vi "Main.vi"() -> ()   [LabVIEW 2017]
panel:
  in  "Sensors Mode":bool
  out "T5":dbl(slide) scale=0.0..150.0
  out "T7":dbl(slide) scale=0.0..150.0
  out "T3":dbl(slide) scale=0.0..150.0
  out "T8":dbl(slide) scale=0.0..150.0
  out "T1":dbl(slide) scale=0.0..150.0
  out "T9":dbl(slide) scale=0.0..150.0
  out "T2":dbl(slide) scale=0.0..150.0
  out "T4":dbl(slide) scale=0.0..150.0
  out "T6":dbl(slide) scale=0.0..150.0
  out "Heater Power":dbl caption="Heater Power P [W]" format="%#.2f"
  out "Heater Temperature":dbl(slide) scale=0.0..250.0
  out "NI2":tag
  out "NI1":tag
  out "Tab Control":enum32{"Page 1", "Page 2"}(tab)
  in  "reset":bool
  in  "Play Button":bool
  out "sec":i16
  out "min":i16
  out "hr":i16
  out "Ky [W/m.K]":dbl
  out "Ks [W/m.K]":dbl
  out "K7-8 [W/m.K]":dbl
  out "K6-7 [W/m.K]":dbl
  out "K5-6 [W/m.K]":dbl
  out "K4-5 [W/m.K]":dbl
  out "K3-4 [W/m.K]":dbl
  out "K2-3 [W/m.K]":dbl
  in  "Exit":bool
  out "X 7 mm":dbl
  out "X 8 mm":dbl
  out "X 9 mm":dbl
  out "X 6 mm":dbl
  out "X 5 mm":dbl
  out "X 4 mm":dbl
  out "X 3 mm":dbl
  out "X 2 mm":dbl
  out "X 1 mm":dbl
  out "K1-2 [W/m.K]":dbl
  out "Heater Temperature T0 [C]":dbl(slide) scale=0.0..250.0
  out "T5 C":dbl(slide) scale=0.0..150.0
  out "T6 C":dbl(slide) scale=0.0..150.0
  out "T4 C":dbl(slide) scale=0.0..150.0
  out "T9 C":dbl(slide) scale=0.0..150.0
  out "T8 C":dbl(slide) scale=0.0..150.0
  out "T7 C":dbl(slide) scale=0.0..150.0
  out "T3 C":dbl(slide) scale=0.0..150.0
  out "T2 C":dbl(slide) scale=0.0..150.0
  out "T1 C":dbl(slide) scale=0.0..150.0
  out "Heater Power linear":dbl caption="Heater Power P [W]" format="%#.2f"
  out "Diameter d [mm]":dbl
  in  "Material Select":string(combo)
  out "Linear Temperature Profile":cluster{"Ramp Pattern":dbl[], dbl[]}[](graph)
  in  "Start Linear":bool
  in  "To Radial":bool
  in  "Save Linear Curve":bool
  in  "Clear Linear Graph":bool
  in  "reset 2":bool
  out "hr 2":i16
  out "min 2":i16
  out "sec 2":i16
  in  "Play Button 2":bool
  out "T45":dbl caption="T45 C" format="%#_5g"
  out "T34":dbl caption="T34 C" format="%#_5g"
  out "T23":dbl caption="T23 C" format="%#_5g"
  out "T12":dbl caption="T12 C" format="%#_5g"
  in  "Exit 2":bool
  out "Thermal Conductivity K [W/m.K]":dbl
  out "T6r":dbl caption="T9 C" format="%#_5g"
  out "T5r":dbl caption="T8 C" format="%#_5g"
  out "T4r":dbl caption="T7 C" format="%#_5g"
  out "T3r":dbl caption="T3 C" format="%#_5g"
  out "T2r":dbl caption="T2 C" format="%#_5g"
  out "T1r":dbl caption="T1 C" format="%#_5g"
  out "Heater Temperature [C]":dbl format="%#_5g"
  out "r1":dbl caption="r1 mm" format="%#_5g"
  out "r2":dbl caption="r2 mm" format="%#_5g"
  out "r3":dbl caption="r3 mm" format="%#_5g"
  out "r4":dbl caption="r4 mm" format="%#_5g"
  out "r5":dbl caption="r5 mm" format="%#_5g"
  out "r6":dbl caption="r6 mm" format="%#_5g"
  out "Radial Temperature Profile":cluster{"Ramp Pattern":dbl[], dbl[]}[](graph)
  in  "To Linear":bool
  in  "Clear Radial Graph":bool
  in  "Save Radial Curve":bool
  out "ri [mm]":dbl caption="Inner Radius ri [mm]"
  out "ro [mm]":dbl caption="Outer Radius ro [mm]"
  out "Disk Thickness [mm]":dbl caption="Disk thinkness t [mm]"
  out "Heater Power rad":dbl caption="Heater Power P [W]"
  in  "Start radial":bool
  # "9"
  # "6"
  # ":"
  # ":"
  # "Linear Experment"
  # "Cooler or heat sink"
  # "Radial Experment"
  # ":"
  # ":"
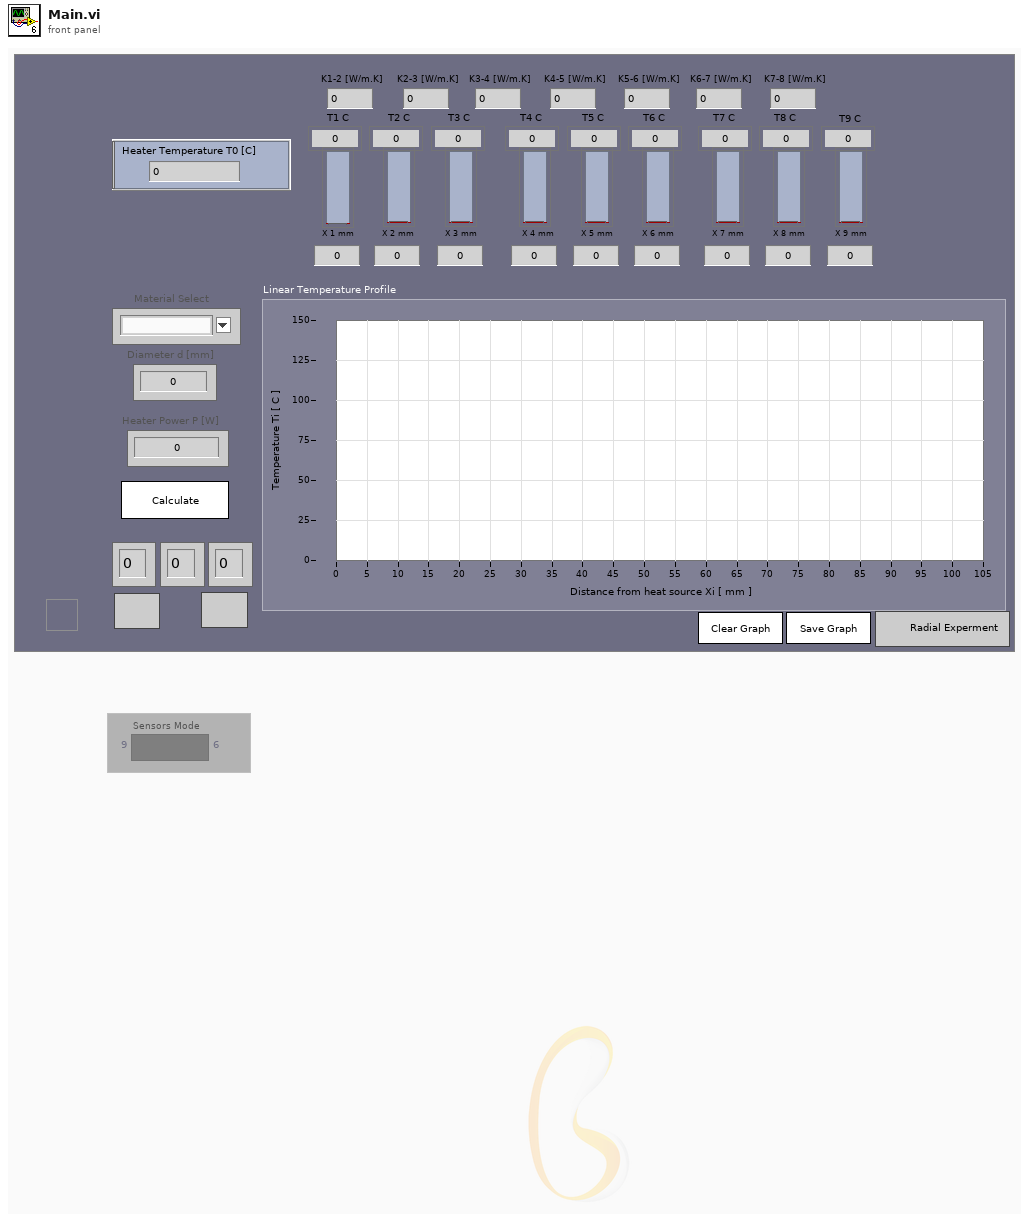
[diagram p1: front panel]
types:
  T1 = enum8{"Enabled", "Disabled", "Disabled and Grayed Out"}
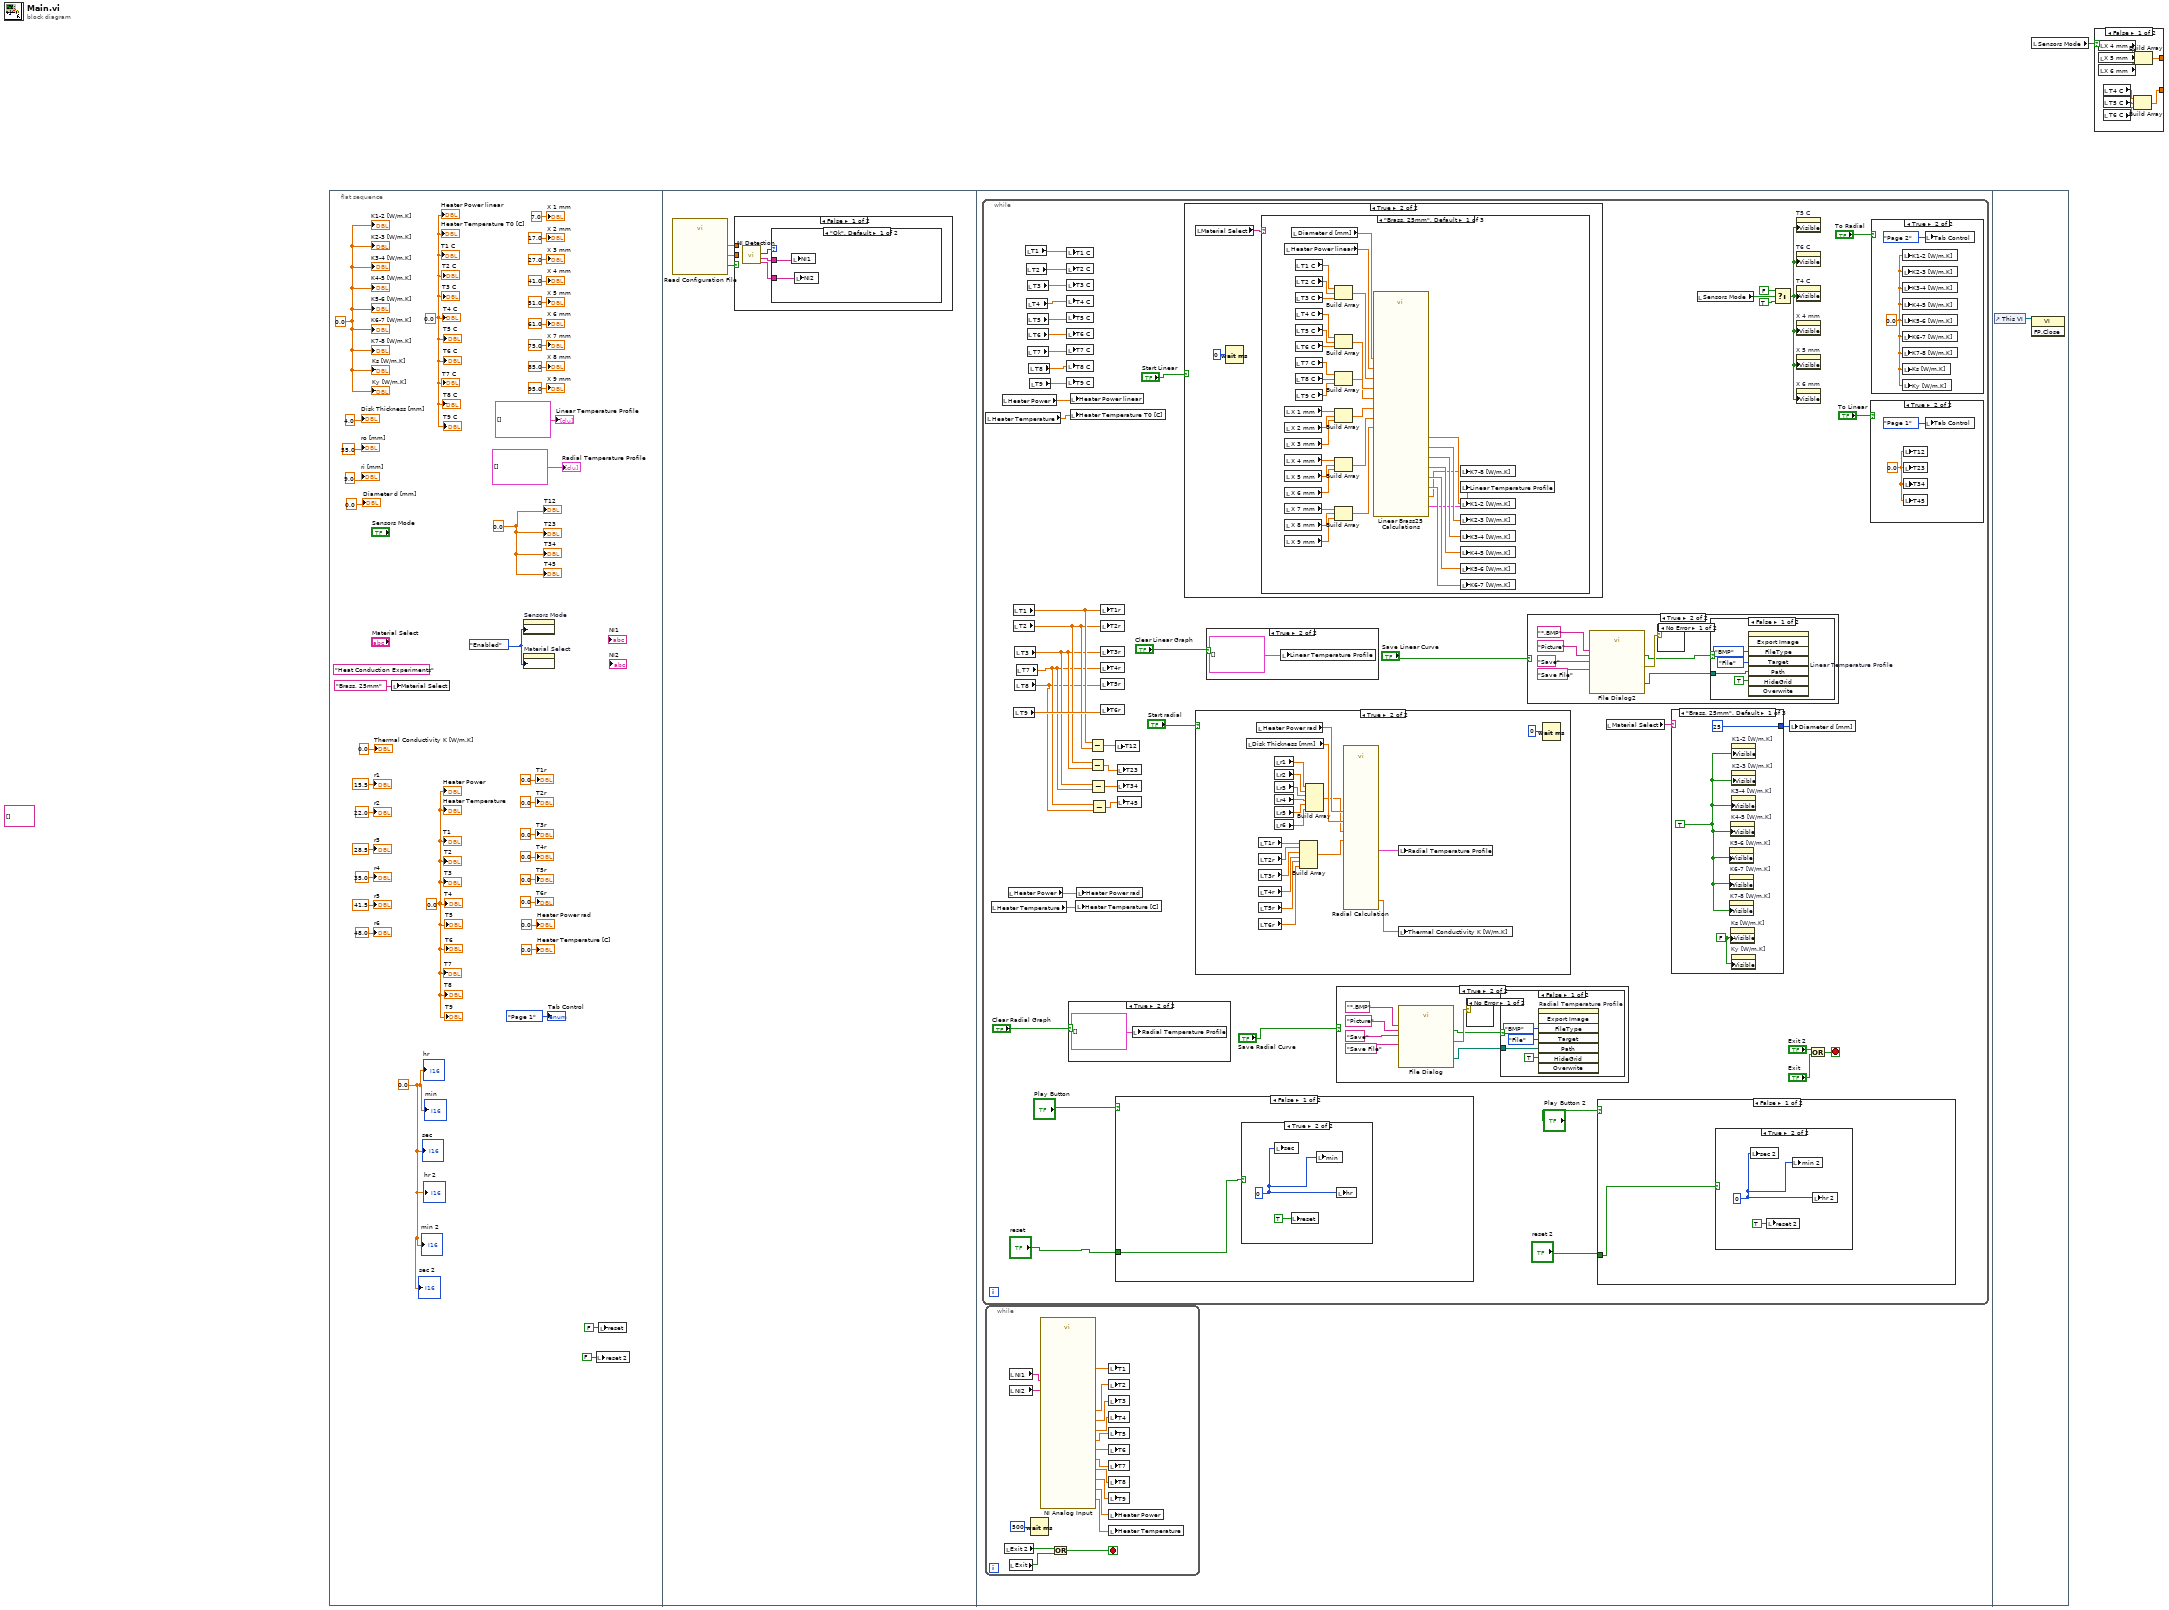
[diagram p0: block diagram]
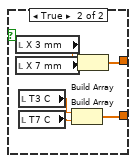
[diagram p2: hidden frame]
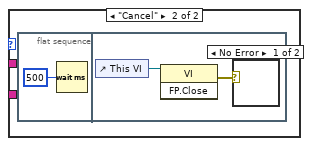
[diagram p3: hidden frame]
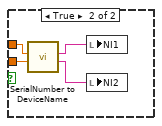
[diagram p5: hidden frame]
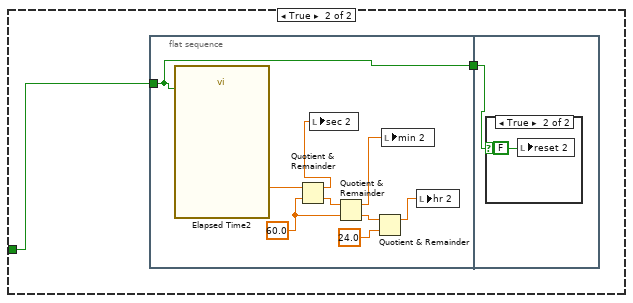
[diagram p7: hidden frame]
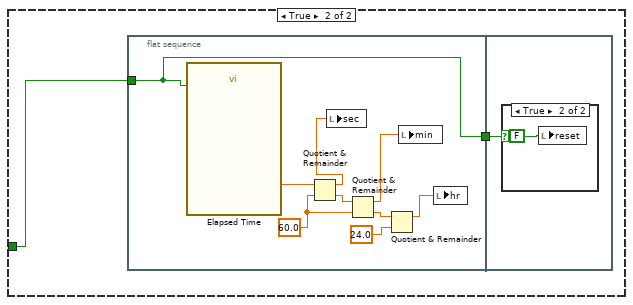
[diagram p10: hidden frame]
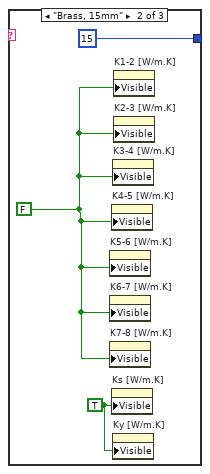
[diagram p14: hidden frame]
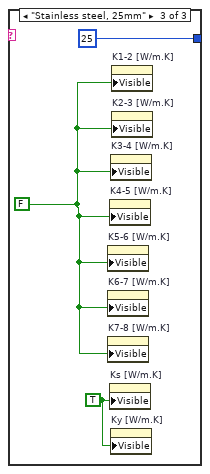
[diagram p15: hidden frame]
diagram:
  (unwired) string[][] [] ("Temperature Table 2")
  n1 = flat-sequence {
    frame #0 {
      w4 = 0.0 ("K")
      w6 = 0.0 ("K1-2 [W/m.K]")
      w5 = 0.0 ("k1- 2")
      w7 = 0.0 ("X1")
      w12 = 0.0 ("X1")
      w36 = T1."Enabled" ("Disabled")
      (unwired) "Heat Conduction Experiments" ("String")
      n2 = local write "Material Select"("Brass, 25mm" ("Material Select")) -> ()
      n3 = property on="Sensors Mode" class="Bool (strict)"("DisabledEnum"=w36) -> ()  [unwired: 2 in, 2 out]
      n4 = property on="Material Select" class="CmbBox"("DisabledEnum"=w36) -> ()  [unwired: 2 in, 2 out]
      n5 = local write "reset 2"(FALSE ("reset 2")) -> ()
      n6 = local write "reset"(FALSE ("reset")) -> ()
      "r3" <- 28.5 ("r3")
      "r2" <- 22.0 ("r2")
      "r1" <- 15.5 ("r1")
      "r4" <- 35.0 ("r4")
      "r5" <- 41.5 ("r5")
      "r6" <- 48.0 ("r6")
      "Heater Power rad" <- 0.0 ("Heater Power rad")
      "Heater Temperature [C]" <- 0.0 ("Heater Temperature")
      "Diameter d [mm]" <- 0.0 ("Diameter d [mm]")
      "ro [mm]" <- 55.0 ("Diameter [mm] radial")
      "Disk Thickness [mm]" <- 4.0 ("Distance [mm] radial")
      "ri [mm]" <- 9.0 ("ri [mm]")
      "X 1 mm" <- 7.0 ("X 1")
      "X 2 mm" <- 17.0 ("X 2")
      "X 3 mm" <- 27.0 ("X 3")
      "X 4 mm" <- 41.0 ("X 4")
      "X 5 mm" <- 51.0 ("X 5")
      "X 6 mm" <- 61.0 ("X 6")
      "X 7 mm" <- 75.0 ("X 7")
      "X 8 mm" <- 85.0 ("X 8")
      "X 9 mm" <- 95.0 ("X 9")
      "Radial Temperature Profile" <- cluster{"Ramp Pattern":dbl[], dbl[]}[] [] ("Temperature Graph radial")
      "Linear Temperature Profile" <- cluster{"Ramp Pattern":dbl[], dbl[]}[] [] ("Linear Temperature Profile")
      "T1r" <- 0.0 ("T1")
      "T2r" <- 0.0 ("T2")
      "T3r" <- 0.0 ("T3")
      "T4r" <- 0.0 ("T4")
      "T5r" <- 0.0 ("T5")
      "T6r" <- 0.0 ("T6")
      "T5 C" <- w12
      "T7 C" <- w12
      "T3 C" <- w12
      "T8 C" <- w12
      "T1 C" <- w12
      "T9 C" <- w12
      "T2 C" <- w12
      "T4 C" <- w12
      "T6 C" <- w12
      "Heater Power linear" <- w12
      "Heater Temperature T0 [C]" <- w12
      "Thermal Conductivity K [W/m.K]" <- 0.0 ("Thermal Conductivity K [W/m.K]")
      "Tab Control" <- enum32{"Page 1", "Page 2"}."Page 1" ("Tab Control")
      "T5" <- w7
      "T7" <- w7
      "T3" <- w7
      "T8" <- w7
      "T1" <- w7
      "T9" <- w7
      "T2" <- w7
      "T4" <- w7
      "T6" <- w7
      "Heater Power" <- w7
      "Heater Temperature" <- w7
      "K2-3 [W/m.K]" <- w6
      "K3-4 [W/m.K]" <- w6
      "K4-5 [W/m.K]" <- w6
      "K5-6 [W/m.K]" <- w6
      "K6-7 [W/m.K]" <- w6
      "K7-8 [W/m.K]" <- w6
      "Ks [W/m.K]" <- w6
      "Ky [W/m.K]" <- w6
      "K1-2 [W/m.K]" <- w6
      "T12" <- w5
      "T23" <- w5
      "T34" <- w5
      "T45" <- w5
      "sec" <- w4
      "min" <- w4
      "hr" <- w4
      "hr 2" <- w4
      "min 2" <- w4
      "sec 2" <- w4
    }
    frame #1 {
      n7 = call "Read Configuration File.vi"() -> ("Serial Numbers Found"=w42:bool, "NI1"=w44:dbl, "NI2"=w43:dbl)  [unwired: 13 in]
      n8 = case shown="False" w42 {
        tunnel: w43 -> [_ w56]
        tunnel: w44 -> [_ w55]
        frame False {
          n9 = call "NI Detection.vi"() -> ("NI 2"=w45:tag, "NI 1"=w46:tag, "Ok/Cancel"=w47:enum16{"Ok", "Cancel"})  [unwired: 8 in]
          n10 = case shown="\"Ok\", Default" w47 {
            tunnel: w46 -> [w49 _]
            tunnel: w45 -> [w48 _]
            frame "Ok", Default {
              n11 = local write "NI1"(w49) -> ()
              n12 = local write "NI2"(w48) -> ()
            }
            frame "Cancel" {
              n13 = flat-sequence {
                frame #0 {
                  n14 = Wait (ms)(milliseconds to wait=u32 500) -> ()  [unwired: 1 out]
                }
                frame #1 {
                  n15 = control-ref of="This VI"() -> (w52:refnum<vi>)
                  n16 = invoke class="VI" method="FP.Close"(reference=w52) -> (error out=w51:errorcluster)  [unwired: 2 in, 2 out]
                  n17 = case shown="No Error" w51 {
                    frame No Error {
                    }
                    frame Error {
                    }
                  }
                }
              }
            }
          }
        }
        frame True {
          n18 = call "SerialNumber to DeviceName.vi"("NI2 Serial Number"=w56, "NI1 Serial Number"=w55) -> ("NI2 Device Name"=w53:tag, "NI1 Device Name"=w54:tag)  [unwired: 8 in]
          n19 = local write "NI1"(w54) -> ()
          n20 = local write "NI2"(w53) -> ()
        }
      }
    }
    frame #2 {
      n21 = while {
        stop <- w103 stop-if-true
        n22 = local read "Heater Temperature"() -> (w102:dbl)
        n23 = local read "Heater Temperature"() -> (w89:dbl)
        n24 = local read "Heater Power"() -> (w101:dbl)
        n25 = local read "Heater Power"() -> (w88:dbl)
        n26 = local read "T1"() -> (w86:dbl)
        n27 = local read "T2"() -> (w85:dbl)
        n28 = local read "T9"() -> (w91:dbl)
        n29 = local read "T3"() -> (w84:dbl)
        n30 = local read "T8"() -> (w82:dbl)
        n31 = local read "T7"() -> (w83:dbl)
        n32 = local read "T1"() -> (w92:dbl)
        n33 = local read "T2"() -> (w93:dbl)
        n34 = local read "T4"() -> (w95:dbl)
        n35 = local read "T3"() -> (w94:dbl)
        n36 = local read "T5"() -> (w96:dbl)
        n37 = local read "T6"() -> (w97:dbl)
        n38 = local read "T7"() -> (w98:dbl)
        n39 = local read "T8"() -> (w99:dbl)
        n40 = local read "T9"() -> (w100:dbl)
        n41 = local write "T1 C"(w92) -> ()
        n42 = local write "T2 C"(w93) -> ()
        n43 = local write "T3 C"(w94) -> ()
        n44 = local write "T4 C"(w95) -> ()
        n45 = local write "T5 C"(w96) -> ()
        n46 = local write "T6 C"(w97) -> ()
        n47 = local write "T7 C"(w98) -> ()
        n48 = local write "T8 C"(w99) -> ()
        n49 = local write "T9 C"(w100) -> ()
        n50 = case shown="True" "Clear Radial Graph" {
          frame False {
          }
          frame True {
            n51 = local write "Radial Temperature Profile"(cluster{"Ramp Pattern":dbl[], dbl[]}[] [] ("Linear Temperature Profile")) -> ()
          }
        }
        n52 = local write "Heater Power linear"(w101) -> ()
        n53 = local write "Heater Temperature T0 [C]"(w102) -> ()
        n54 = local write "Heater Temperature [C]"(w89) -> ()
        n55 = local write "Heater Power rad"(w88) -> ()
        n56 = Subtract(x=w86, y=w85) -> (x-y=w81:dbl)
        n57 = Subtract(x=w85, y=w84) -> (x-y=w80:dbl)
        n58 = Subtract(x=w84, y=w83) -> (x-y=w79:dbl)
        n59 = Subtract(x=w83, y=w82) -> (x-y=w78:dbl)
        n60 = local write "T1r"(w86) -> ()
        n61 = local write "T2r"(w85) -> ()
        n62 = local write "T3r"(w84) -> ()
        n63 = local write "T4r"(w83) -> ()
        n64 = local write "T5r"(w82) -> ()
        n65 = local write "T6r"(w91) -> ()
        n66 = local write "T12"(w81) -> ()
        n67 = case shown="False" "Play Button" {
          tunnel: "reset" -> [w134 w138]
          frame False {
            n68 = case shown="True" w134 {
              frame False {
              }
              frame True {
                w136 = i16 0 ("sec")
                n69 = local write "sec"(w136) -> ()
                n70 = local write "reset"(TRUE ("reset")) -> ()
                n71 = local write "min"(w136) -> ()
                n72 = local write "hr"(w136) -> ()
              }
            }
          }
          frame True {
            n73 = flat-sequence {
              tunnel: w138 -> [w139]
              tunnel: [w139] -> w137
              tunnel: w137 -> [w148]
              frame #0 {
                w142 = 60.0 ("y")
                n74 = call "Elapsed Time"("Reset"=w139) -> ("Elapsed Time (s)"=w140:dbl)  [unwired: 11 in, 7 out]
                n75 = Quotient & Remainder(x=w140, y=w142) -> (x-y*floor(x/y)=w143:dbl, floor(x/y)=w147:dbl)
                n76 = local write "sec"(w143) -> ()
                n77 = Quotient & Remainder(x=w147, y=w142) -> (x-y*floor(x/y)=w144:dbl, floor(x/y)=w146:dbl)
                n78 = Quotient & Remainder(x=w146, y=24.0) -> (x-y*floor(x/y)=w145:dbl)  [unwired: 1 out]
                n79 = local write "min"(w144) -> ()
                n80 = local write "hr"(w145) -> ()
              }
              frame #1 {
                n81 = case shown="True" w148 {
                  frame False {
                  }
                  frame True {
                    n82 = local write "reset"(FALSE ("reset")) -> ()
                  }
                }
              }
            }
          }
        }
        n83 = local write "T23"(w80) -> ()
        n84 = local write "T34"(w79) -> ()
        n85 = local write "T45"(w78) -> ()
        n86 = case shown="True" "Start Linear" {
          frame False {
          }
          frame True {
            n87 = local read "Material Select"() -> (w207:string)
            n88 = Wait (ms)(milliseconds to wait=u32 0) -> ()  [unwired: 1 out]
            n89 = case shown="\"Brass, 25mm\", Default" w207 {
              frame "Brass, 25mm", Default {
                n90 = local read "Heater Power linear"() -> (w222:dbl)
                n91 = local read "X 1 mm"() -> (w238:dbl)
                n92 = local read "X 2 mm"() -> (w237:dbl)
                n93 = local read "X 3 mm"() -> (w236:dbl)
                n94 = local read "X 4 mm"() -> (w226:dbl)
                n95 = local read "X 5 mm"() -> (w225:dbl)
                n96 = local read "X 6 mm"() -> (w224:dbl)
                n97 = local read "X 7 mm"() -> (w239:dbl)
                n98 = local read "X 8 mm"() -> (w240:dbl)
                n99 = local read "X 9 mm"() -> (w241:dbl)
                n100 = local read "Diameter d [mm]"() -> (w223:dbl)
                n101 = local read "T1 C"() -> (w230:dbl)
                n102 = local read "T2 C"() -> (w231:dbl)
                n103 = local read "T3 C"() -> (w232:dbl)
                n104 = local read "T4 C"() -> (w229:dbl)
                n105 = local read "T5 C"() -> (w228:dbl)
                n106 = local read "T6 C"() -> (w227:dbl)
                n107 = local read "T7 C"() -> (w235:dbl)
                n108 = local read "T8 C"() -> (w234:dbl)
                n109 = local read "T9 C"() -> (w233:dbl)
                n110 = Build Array(w230, w231, w232) -> (w221:dbl[])
                n111 = Build Array(w229, w228, w227) -> (w220:dbl[])
                n112 = Build Array(w235, w234, w233) -> (w219:dbl[])
                n113 = Build Array(w238, w237, w236) -> (w218:dbl[])
                n114 = Build Array(w226, w225, w224) -> (w217:dbl[])
                n115 = Build Array(w239, w240, w241) -> (w216:dbl[])
                n116 = call "Linear Brass25 Calculations.vi"("Power"=w222, "Diameter"=w223, "X1"=w218, "T1"=w221, "X2"=w217, "T2"=w220, "X3"=w216, "T3"=w219) -> ("K1-2"=w215:dbl, "K2-3"=w214:dbl, "K3-4"=w213:dbl, "K4-5"=w212:dbl, "XY Graph"=w208:cluster{"Ramp Pattern":dbl[], dbl[]}[], "K5-6"=w211:dbl, "K6-7"=w210:dbl, "K7-8"=w209:dbl)  [unwired: 12 in]
                n117 = local write "K7-8 [W/m.K]"(w209) -> ()
                n118 = local write "Linear Temperature Profile"(w208) -> ()
                n119 = local write "K1-2 [W/m.K]"(w215) -> ()
                n120 = local write "K2-3 [W/m.K]"(w214) -> ()
                n121 = local write "K3-4 [W/m.K]"(w213) -> ()
                n122 = local write "K4-5 [W/m.K]"(w212) -> ()
                n123 = local write "K5-6 [W/m.K]"(w211) -> ()
                n124 = local write "K6-7 [W/m.K]"(w210) -> ()
              }
              frame "Brass, 15mm" {
                n125 = local read "Heater Power linear"() -> (w244:dbl)
                n126 = local read "T1 C"() -> (w259:dbl)
                n127 = local read "T2 C"() -> (w260:dbl)
                n128 = local read "T3 C"() -> (w261:dbl)
                n129 = local read "T7 C"() -> (w257:dbl)
                n130 = local read "T8 C"() -> (w256:dbl)
                n131 = local read "T9 C"() -> (w255:dbl)
                n132 = local read "X 1 mm"() -> (w253:dbl)
                n133 = local read "X 2 mm"() -> (w252:dbl)
                n134 = local read "X 3 mm"() -> (w251:dbl)
                n135 = local read "X 7 mm"() -> (w247:dbl)
                n136 = local read "X 8 mm"() -> (w248:dbl)
                n137 = local read "X 9 mm"() -> (w249:dbl)
                n138 = Build Array(w259, w260, w261) -> (w258:dbl[])
                n139 = Build Array(w257, w256, w255) -> (w254:dbl[])
                n140 = Build Array(w253, w252, w251) -> (w250:dbl[])
                n141 = Build Array(w247, w248, w249) -> (w246:dbl[])
                n142 = call "Linear Brass15 Calculations.vi"("Power"=w244, "X1"=w250, "T1"=w258, "X3"=w246, "T3"=w254) -> ("Ks"=w242:dbl, "Ky"=w243:dbl, "XY Graph"=w245:cluster{"Ramp Pattern":dbl[], dbl[]}[])  [unwired: 20 in]
                n143 = local write "Linear Temperature Profile"(w245) -> ()
                n144 = local write "Ks [W/m.K]"(w242) -> ()
                n145 = local write "Ky [W/m.K]"(w243) -> ()
              }
              frame "Stainless steel, 25mm" {
                n146 = local read "Heater Power linear"() -> (w269:dbl)
                n147 = local read "T1 C"() -> (w279:dbl)
                n148 = local read "T2 C"() -> (w280:dbl)
                n149 = local read "T3 C"() -> (w281:dbl)
                n150 = local read "T7 C"() -> (w278:dbl)
                n151 = local read "T8 C"() -> (w277:dbl)
                n152 = local read "T9 C"() -> (w276:dbl)
                n153 = local read "X 1 mm"() -> (w275:dbl)
                n154 = local read "X 2 mm"() -> (w274:dbl)
                n155 = local read "X 3 mm"() -> (w273:dbl)
                n156 = local read "X 7 mm"() -> (w270:dbl)
                n157 = local read "X 8 mm"() -> (w271:dbl)
                n158 = local read "X 9 mm"() -> (w272:dbl)
                n159 = Build Array(w279, w280, w281) -> (w268:dbl[])
                n160 = Build Array(w278, w277, w276) -> (w267:dbl[])
                n161 = Build Array(w275, w274, w273) -> (w266:dbl[])
                n162 = Build Array(w270, w271, w272) -> (w265:dbl[])
                n163 = call "Linear stainless25 Calculations.vi"("Power"=w269, "X1"=w266, "T1"=w268, "X3"=w265, "T3"=w267) -> ("Ks"=w262:dbl, "Ky"=w263:dbl, "XY Graph"=w264:cluster{"Ramp Pattern":dbl[], dbl[]}[])  [unwired: 20 in]
                n164 = local write "Linear Temperature Profile"(w264) -> ()
                n165 = local write "Ks [W/m.K]"(w262) -> ()
                n166 = local write "Ky [W/m.K]"(w263) -> ()
              }
            }
          }
        }
        n167 = case shown="True" "Start radial" {
          frame False {
          }
          frame True {
            n168 = local read "Disk Thickness [mm]"() -> (w204:dbl)
            n169 = local read "Heater Power rad"() -> (w205:dbl)
            n170 = local read "T1r"() -> (w203:dbl)
            n171 = local read "T2r"() -> (w202:dbl)
            n172 = local read "T3r"() -> (w201:dbl)
            n173 = local read "T4r"() -> (w200:dbl)
            n174 = local read "T5r"() -> (w199:dbl)
            n175 = local read "T6r"() -> (w198:dbl)
            n176 = local read "r1"() -> (w192:dbl)
            n177 = local read "r2"() -> (w193:dbl)
            n178 = local read "r3"() -> (w194:dbl)
            n179 = local read "r4"() -> (w195:dbl)
            n180 = local read "r5"() -> (w196:dbl)
            n181 = local read "r6"() -> (w197:dbl)
            n182 = Build Array(w203, w202, w201, w200, w199, w198) -> (w190:dbl[])
            n183 = Build Array(w192, w193, w194, w195, w196, w197) -> (w191:dbl[])
            n184 = call "Radial Calculation.vi"("Power"=w205, "X"=w191, "Thikness"=w204, "Y"=w190) -> ("XY Graph"=w189:cluster{"Ramp Pattern":dbl[], dbl[]}[], "Result"=w187:dbl)  [unwired: 6 in, 4 out]
            n185 = local write "Radial Temperature Profile"(w189) -> ()
            n186 = local write "Thermal Conductivity K [W/m.K]"(w187) -> ()
            n187 = Wait (ms)(milliseconds to wait=u32 0) -> ()  [unwired: 1 out]
          }
        }
        n188 = case shown="True" "Clear Linear Graph" {
          frame False {
          }
          frame True {
            n189 = local write "Linear Temperature Profile"(cluster{"Ramp Pattern":dbl[], dbl[]}[] [] ("Linear Temperature Profile")) -> ()
          }
        }
        n190 = case shown="True" "Save Radial Curve" {
          frame False {
          }
          frame True {
            n191 = call "File Dialog"("prompt"="Save File", "button label"="Save", "pattern (all files)"="*.BMP", "pattern label"="Picture") -> ("selected path"=w163:path, "cancelled"=w164:bool, "error out"=w169:errorcluster)  [unwired: 8 in, 1 out]
            n192 = case shown="No Error" w169 {
              frame No Error {
              }
              frame Error {
              }
            }
            n193 = case shown="False" w164 {
              tunnel: w163 -> [w170 _]
              frame False {
                n194 = invoke on="Radial Temperature Profile" class="XYGraph (strict)" method="Export Image"("FileType"=enum32{"BMP", "EPS", "EMF", "PICT"}."BMP" ("File Type"), "Target"=enum32{"File", "Clipboard"}."File", "Path"=w170, "HideGrid"=TRUE ("Hide Grid")) -> ()  [unwired: 4 in, 8 out]
              }
              frame True {
              }
            }
          }
        }
        n195 = case shown="True" "Save Linear Curve" {
          frame False {
          }
          frame True {
            n196 = call "File Dialog2"("prompt"="Save File", "button label"="Save", "pattern (all files)"="*.BMP", "pattern label"="Picture") -> ("selected path"=w175:path, "cancelled"=w176:bool, "error out"=w177:errorcluster)  [unwired: 8 in, 1 out]
            n197 = case shown="No Error" w177 {
              frame No Error {
              }
              frame Error {
              }
            }
            n198 = case shown="False" w176 {
              tunnel: w175 -> [w182 _]
              frame False {
                n199 = invoke on="Linear Temperature Profile" class="XYGraph (strict)" method="Export Image"("FileType"=enum32{"BMP", "EPS", "EMF", "PICT"}."BMP" ("File Type"), "Target"=enum32{"File", "Clipboard"}."File", "Path"=w182, "HideGrid"=TRUE ("Hide Grid")) -> ()  [unwired: 4 in, 8 out]
              }
              frame True {
              }
            }
          }
        }
        n200 = case shown="False" "Play Button 2" {
          tunnel: "reset 2" -> [w118 w122]
          frame False {
            n201 = case shown="True" w118 {
              frame False {
              }
              frame True {
                w119 = i16 0 ("sec")
                n202 = local write "sec 2"(w119) -> ()
                n203 = local write "reset 2"(TRUE ("reset")) -> ()
                n204 = local write "min 2"(w119) -> ()
                n205 = local write "hr 2"(w119) -> ()
              }
            }
          }
          frame True {
            n206 = flat-sequence {
              tunnel: w122 -> [w123]
              tunnel: [w123] -> w121
              tunnel: w121 -> [w132]
              frame #0 {
                w126 = 60.0 ("y")
                n207 = call "Elapsed Time2"("Reset"=w123) -> ("Elapsed Time (s)"=w124:dbl)  [unwired: 11 in, 7 out]
                n208 = Quotient & Remainder(x=w124, y=w126) -> (x-y*floor(x/y)=w127:dbl, floor(x/y)=w131:dbl)
                n209 = local write "sec 2"(w127) -> ()
                n210 = Quotient & Remainder(x=w131, y=w126) -> (x-y*floor(x/y)=w128:dbl, floor(x/y)=w130:dbl)
                n211 = Quotient & Remainder(x=w130, y=24.0) -> (x-y*floor(x/y)=w129:dbl)  [unwired: 1 out]
                n212 = local write "min 2"(w128) -> ()
                n213 = local write "hr 2"(w129) -> ()
              }
              frame #1 {
                n214 = case shown="True" w132 {
                  frame False {
                  }
                  frame True {
                    n215 = local write "reset 2"(FALSE ("reset")) -> ()
                  }
                }
              }
            }
          }
        }
        n216 = local read "Material Select"() -> (w108:string)
        n217 = case shown="\"Brass, 25mm\", Default" w108 {
          tunnel: [25 15 25] -> w109
          frame "Brass, 25mm", Default {
            w154 = FALSE ("Visible")
            w155 = TRUE ("Visible")
            n218 = property on="K5-6 [W/m.K]" class="DigNum (strict)"("Visible"=w155) -> ()  [unwired: 2 in, 2 out]
            n219 = property on="K6-7 [W/m.K]" class="DigNum (strict)"("Visible"=w155) -> ()  [unwired: 2 in, 2 out]
            n220 = property on="K7-8 [W/m.K]" class="DigNum (strict)"("Visible"=w155) -> ()  [unwired: 2 in, 2 out]
            n221 = property on="K4-5 [W/m.K]" class="DigNum (strict)"("Visible"=w155) -> ()  [unwired: 2 in, 2 out]
            n222 = property on="Ks [W/m.K]" class="DigNum (strict)"("Visible"=w154) -> ()  [unwired: 2 in, 2 out]
            n223 = property on="K3-4 [W/m.K]" class="DigNum (strict)"("Visible"=w155) -> ()  [unwired: 2 in, 2 out]
            n224 = property on="Ky [W/m.K]" class="DigNum (strict)"("Visible"=w154) -> ()  [unwired: 2 in, 2 out]
            n225 = property on="K1-2 [W/m.K]" class="DigNum (strict)"("Visible"=w155) -> ()  [unwired: 2 in, 2 out]
            n226 = property on="K2-3 [W/m.K]" class="DigNum (strict)"("Visible"=w155) -> ()  [unwired: 2 in, 2 out]
          }
          frame "Brass, 15mm" {
            w157 = TRUE ("Visible")
            w158 = FALSE ("Visible")
            n227 = property on="K5-6 [W/m.K]" class="DigNum (strict)"("Visible"=w158) -> ()  [unwired: 2 in, 2 out]
            n228 = property on="K6-7 [W/m.K]" class="DigNum (strict)"("Visible"=w158) -> ()  [unwired: 2 in, 2 out]
            n229 = property on="K7-8 [W/m.K]" class="DigNum (strict)"("Visible"=w158) -> ()  [unwired: 2 in, 2 out]
            n230 = property on="K4-5 [W/m.K]" class="DigNum (strict)"("Visible"=w158) -> ()  [unwired: 2 in, 2 out]
            n231 = property on="Ks [W/m.K]" class="DigNum (strict)"("Visible"=w157) -> ()  [unwired: 2 in, 2 out]
            n232 = property on="K3-4 [W/m.K]" class="DigNum (strict)"("Visible"=w158) -> ()  [unwired: 2 in, 2 out]
            n233 = property on="Ky [W/m.K]" class="DigNum (strict)"("Visible"=w157) -> ()  [unwired: 2 in, 2 out]
            n234 = property on="K1-2 [W/m.K]" class="DigNum (strict)"("Visible"=w158) -> ()  [unwired: 2 in, 2 out]
            n235 = property on="K2-3 [W/m.K]" class="DigNum (strict)"("Visible"=w158) -> ()  [unwired: 2 in, 2 out]
          }
          frame "Stainless steel, 25mm" {
            w160 = TRUE ("Visible")
            w161 = FALSE ("Visible")
            n236 = property on="K5-6 [W/m.K]" class="DigNum (strict)"("Visible"=w161) -> ()  [unwired: 2 in, 2 out]
            n237 = property on="K6-7 [W/m.K]" class="DigNum (strict)"("Visible"=w161) -> ()  [unwired: 2 in, 2 out]
            n238 = property on="K7-8 [W/m.K]" class="DigNum (strict)"("Visible"=w161) -> ()  [unwired: 2 in, 2 out]
            n239 = property on="K4-5 [W/m.K]" class="DigNum (strict)"("Visible"=w161) -> ()  [unwired: 2 in, 2 out]
            n240 = property on="Ks [W/m.K]" class="DigNum (strict)"("Visible"=w160) -> ()  [unwired: 2 in, 2 out]
            n241 = property on="K3-4 [W/m.K]" class="DigNum (strict)"("Visible"=w161) -> ()  [unwired: 2 in, 2 out]
            n242 = property on="Ky [W/m.K]" class="DigNum (strict)"("Visible"=w160) -> ()  [unwired: 2 in, 2 out]
            n243 = property on="K1-2 [W/m.K]" class="DigNum (strict)"("Visible"=w161) -> ()  [unwired: 2 in, 2 out]
            n244 = property on="K2-3 [W/m.K]" class="DigNum (strict)"("Visible"=w161) -> ()  [unwired: 2 in, 2 out]
          }
        }
        n245 = local read "Sensors Mode"() -> (w110:bool)
        n246 = Select(t=FALSE ("Visible"), s=w110, f=TRUE ("Visible")) -> (s? t:f=w111:bool)
        n247 = local write "Diameter d [mm]"(w109) -> ()
        n248 = property on="T5 C" class="Slide (strict)"("Visible"=w111) -> ()  [unwired: 2 in, 2 out]
        n249 = property on="T6 C" class="Slide (strict)"("Visible"=w111) -> ()  [unwired: 2 in, 2 out]
        n250 = property on="T4 C" class="Slide (strict)"("Visible"=w111) -> ()  [unwired: 2 in, 2 out]
        n251 = property on="X 4 mm" class="DigNum (strict)"("Visible"=w111) -> ()  [unwired: 2 in, 2 out]
        n252 = property on="X 5 mm" class="DigNum (strict)"("Visible"=w111) -> ()  [unwired: 2 in, 2 out]
        n253 = property on="X 6 mm" class="DigNum (strict)"("Visible"=w111) -> ()  [unwired: 2 in, 2 out]
        n254 = Or(x="Exit 2", y="Exit") -> (x .or. y?=w103:bool)
        n255 = case shown="True" "To Linear" {
          frame False {
          }
          frame True {
            w150 = 0.0 ("k2- 3")
            n256 = local write "T12"(w150) -> ()
            n257 = local write "T23"(w150) -> ()
            n258 = local write "T34"(w150) -> ()
            n259 = local write "T45"(w150) -> ()
            n260 = local write "Tab Control"(enum32{"Page 1", "Page 2"}."Page 1" ("Tab Control")) -> ()
          }
        }
        n261 = case shown="True" "To Radial" {
          frame False {
          }
          frame True {
            w152 = 0.0 ("T6")
            n262 = local write "K1-2 [W/m.K]"(w152) -> ()
            n263 = local write "K2-3 [W/m.K]"(w152) -> ()
            n264 = local write "K3-4 [W/m.K]"(w152) -> ()
            n265 = local write "K4-5 [W/m.K]"(w152) -> ()
            n266 = local write "K5-6 [W/m.K]"(w152) -> ()
            n267 = local write "K6-7 [W/m.K]"(w152) -> ()
            n268 = local write "K7-8 [W/m.K]"(w152) -> ()
            n269 = local write "Ks [W/m.K]"(w152) -> ()
            n270 = local write "Ky [W/m.K]"(w152) -> ()
            n271 = local write "Tab Control"(enum32{"Page 1", "Page 2"}."Page 2" ("Tab Control")) -> ()
          }
        }
      }
      n272 = while {
        stop <- w68 stop-if-true
        n273 = local read "Exit 2"() -> (w69:bool)
        n274 = local read "NI1"() -> (w73:tag)
        n275 = local read "NI2"() -> (w72:tag)
        n276 = local read "Exit"() -> (w70:bool)
        n277 = Wait (ms)(milliseconds to wait=u32 500) -> ()  [unwired: 1 out]
        n278 = call "NI Analog Input.vi"("NI1"=w73, "NI2"=w72) -> ("T1"=w67:dbl, "T2"=w66:dbl, "T3"=w65:dbl, "T4"=w64:dbl, "T5"=w63:dbl, "T6"=w62:dbl, "T7"=w61:dbl, "T8"=w60:dbl, "T9"=w59:dbl, "Heater Temp"=w57:dbl, "Heater Power"=w58:dbl)  [unwired: 15 in]
        n279 = Or(x=w69, y=w70) -> (x .or. y?=w68:bool)
        n280 = local write "T1"(w67) -> ()
        n281 = local write "T2"(w66) -> ()
        n282 = local write "T3"(w65) -> ()
        n283 = local write "T4"(w64) -> ()
        n284 = local write "T5"(w63) -> ()
        n285 = local write "T6"(w62) -> ()
        n286 = local write "T7"(w61) -> ()
        n287 = local write "T8"(w60) -> ()
        n288 = local write "T9"(w59) -> ()
        n289 = local write "Heater Power"(w58) -> ()
        n290 = local write "Heater Temperature"(w57) -> ()
      }
    }
    frame #3 {
      n291 = control-ref of="This VI"() -> (w282:refnum<vi>)
      n292 = invoke class="VI" method="FP.Close"(reference=w282) -> ()  [unwired: 2 in, 3 out]
    }
  }
  n293 = local read "Sensors Mode"() -> (w1:bool)
  n294 = case shown="False" w1 {
    tunnel: [w284 w292] -> _
    tunnel: [w283 w291] -> _
    frame False {
      n295 = local read "X 4 mm"() -> (w288:dbl)
      n296 = local read "X 5 mm"() -> (w289:dbl)
      n297 = local read "X 6 mm"() -> (w290:dbl)
      n298 = local read "T4 C"() -> (w285:dbl)
      n299 = local read "T5 C"() -> (w286:dbl)
      n300 = local read "T6 C"() -> (w287:dbl)
      n301 = Build Array(w285, w286, w287) -> (w283:dbl[])
      n302 = Build Array(w288, w289, w290) -> (w284:dbl[])
    }
    frame True {
      n303 = local read "X 3 mm"() -> (w293:dbl)
      n304 = local read "X 7 mm"() -> (w294:dbl)
      n305 = local read "T3 C"() -> (w295:dbl)
      n306 = local read "T7 C"() -> (w296:dbl)
      n307 = Build Array(w295, w296) -> (w291:dbl[])
      n308 = Build Array(w293, w294) -> (w292:dbl[])
    }
  }
